vi "Bool to u8.vi"(11 "Input":bool[](array[boolean])) -> (3 "Output":u8 format="%08b")   [LabVIEW 2025, in "TD4.lvclass"]
uses:
  TD4.lvclass
  TD4.lvclass/TD4.ctl
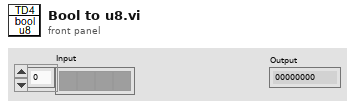
[diagram p1: front panel]
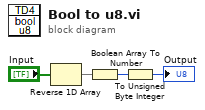
[diagram p0: block diagram]
diagram:
  n1 = Reverse 1D Array(array="Input") -> (reversed array=w3:bool[])
  n2 = Boolean Array To Number(Boolean array=w3) -> (number=w2:u32)
  n3 = To Unsigned Byte Integer(number=w2) -> (unsigned 8bit integer=→"Output":u8)
